vi "Is Null.vi"(1 "Deserialized JSON Data":variant) -> (0 "Null?":bool)   [LabVIEW 2013, in "JKI JSON Serialization.lvlib"]
uses:
  JKI JSON Serialization.lvlib
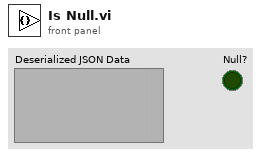
[diagram p1: front panel]
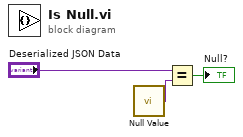
[diagram p0: block diagram]
diagram:
  n1 = call "Null Value.vi"() -> ("Null"=w2:variant)
  n2 = Equal?(x="Deserialized JSON Data", y=w2) -> (x = y?=→"Null?":bool)
